vi "Read Settings File.vi"(8 "error in (no error)":errorcluster) -> (0 "error out":errorcluster, 3 "Settings":T1={"LCR VISA Resource"="", "PSU VISA Resource"="", "AI Task"="AI_Task", "AO Task"="AO_Task", "DO Task"="DO_Task", "Report Directory"=path ""})   [LabVIEW 2018]
uses:
  controls/Settings.ctl
  53bc5963-49c2-488d-b7ac-7ebb16c4e733.vi
  <vilib>/JDP Science/JSONtext/JSON text to Variant.vi
  <vilib>/JDP Science/JSONtext/LVClass Serializer/JSONtext LVClass Serializer.lvclass
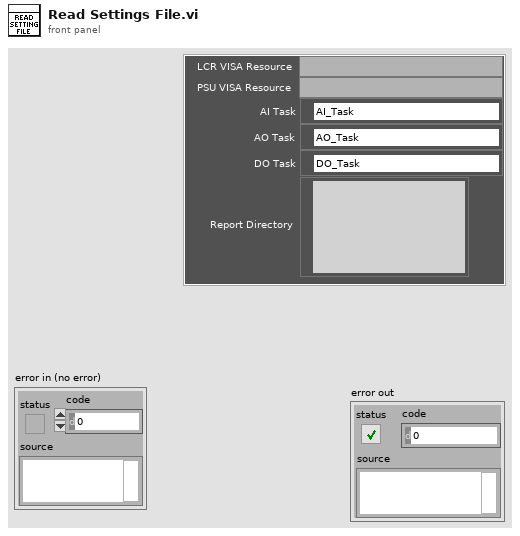
[diagram p1: front panel]
types:
  T1 = typedef "Settings.ctl" = cluster{"LCR VISA Resource":refnum<visa-resource-name>, "PSU VISA Resource":refnum<visa-resource-name>, "AI Task":refnum<k21>, "AO Task":refnum<k21>, "DO Task":refnum<k21>, "Report Directory":path}
  T2 = enum16{"open", "replace", "create", "open or create", "replace or create", "replace or create with confirmation"}
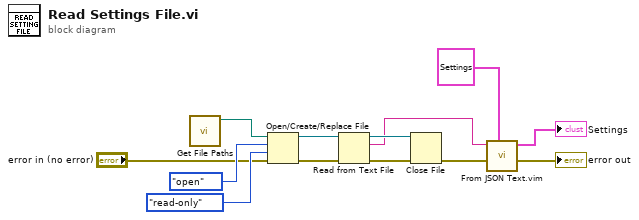
[diagram p0: block diagram]
diagram:
  n1 = call "Get File Paths.vi"() -> ("Settings Path"=w13:path)  [unwired: 10 in, 1 out]
  n2 = Open/Create/Replace File(file path (use dialog)=w13, error in="error in (no error)", operation (0:open)=T2."open", access (0:read/write)=enum16{"read/write", "read-only", "write-only"}."read-only") -> (refnum out=w9:refnum<file>, error out=w10:errorcluster)  [unwired: 2 in, 1 out]
  n3 = Read from Text File(file (use dialog)=w9, error in=w10) -> (refnum out=w7:refnum<file>, text=w2:string, error out=w8:errorcluster)  [unwired: 2 in, 1 out]
  n4 = Close File(refnum=w7, error in=w8) -> (error out=w5:errorcluster)  [unwired: 1 out]
  n5 = call "From JSON Text.vim"("Data Type and Default Value"=T1 {"LCR VISA Resource"="", "PSU VISA Resource"="", "AI Task"="AI_Task", "AO Task"="AO_Task", "DO Task"="DO_Task", "Report Directory"=path ""} ("Settings"), "error in (no error)"=w5, "JSON"=w2) -> ("error out"=→"error out":errorcluster, "Data out"=→"Settings":T1)  [unwired: 7 in]
